vi "VISA_GPIB_TEST.vi"() -> ()   [LabVIEW 2015]
panel:
  out "Raw Data":string
  in  "VISA resource name":refnum<visa-resource-name>
  in  "VISA Open timeout (0)":u32
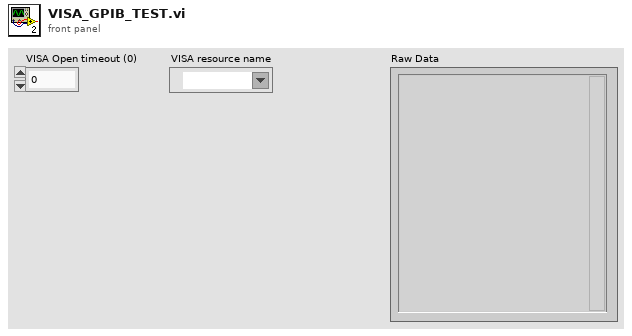
[diagram p1: front panel]
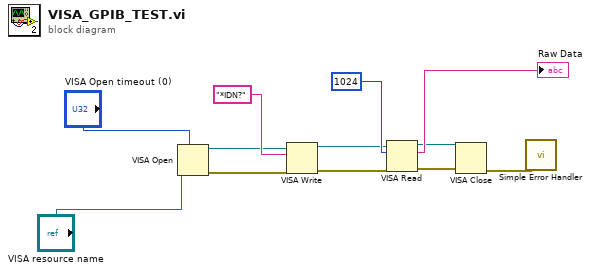
[diagram p0: block diagram]
diagram:
  n1 = VISA Open(timeout (0)="VISA Open timeout (0)", VISA resource name="VISA resource name") -> (VISA resource name=w9:refnum<visa-resource-name>, error out=w8:errorcluster)  [unwired: 3 in]
  n2 = VISA Write(VISA resource name=w9, write buffer="*IDN?", error in (no error)=w8) -> (VISA resource name out=w6:refnum<visa-resource-name>, error out=w5:errorcluster)  [unwired: 1 out]
  n3 = VISA Read(VISA resource name=w6, byte count=u32 1024, error in (no error)=w5) -> (VISA resource name out=w3:refnum<visa-resource-name>, read buffer=→"Raw Data":string, error out=w2:errorcluster)  [unwired: 1 out]
  n4 = VISA Close(VISA resource name=w3, error in (no error)=w2) -> (error out=w1:errorcluster)
  n5 = call <vilib>:"Simple Error Handler.vi"("error in (no error)"=w1) -> ()  [unwired: 4 in, 5 out]
